vi "_API_BINANCE_DELETE_CanelAllOpenOrderOnASymbol.vi"(0 "BinanceAPI_.lvclass":refnum<class "BinanceAPI_.lvclass">, 5 "CanelAllOpenOrderOnSymbol":T1={"symbol (BTCUSDT)"="CAKEUSDT", "recvWindow"=5000}, 11 "error in (no error)":errorcluster) -> (4 "BinanceAPI_.lvclass 2":refnum<class "BinanceAPI_.lvclass">, 14 "Body":string, 15 "error out":errorcluster)   [LabVIEW 2022 SP3, in "BinanceAPI_.lvclass"]
doc: "Delete all open orders on symbol"
uses:
  BinanceAPI_.lvclass
  BinanceAPI_.lvclass/BinanceAPI_.ctl
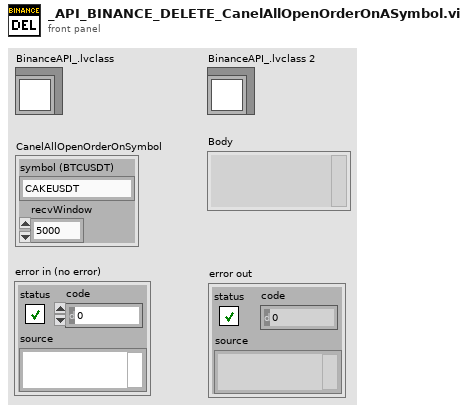
[diagram p1: front panel]
types:
  T1 = cluster{"symbol (BTCUSDT)":string, "recvWindow":i32}
  T2 = enum16{"SPOT", "USDT_FUTURES", "COIN_FUTURES", "VANILLA"}
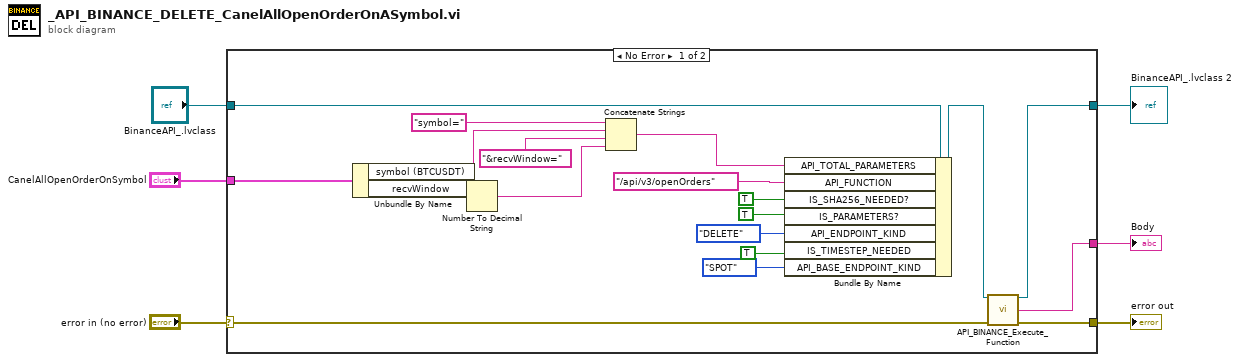
[diagram p0: block diagram]
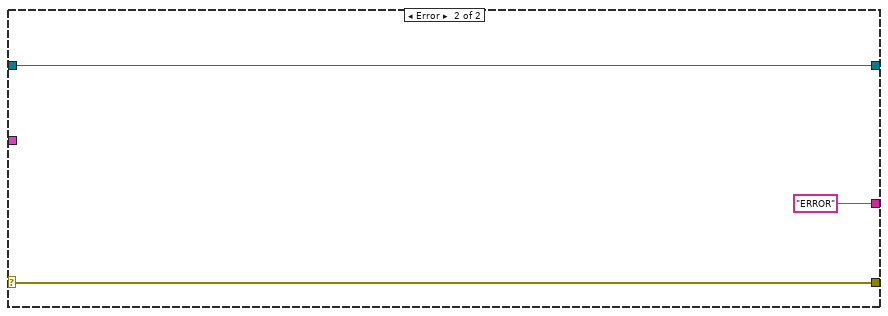
[diagram p2: hidden frame]
diagram:
  n1 = case shown="No Error" "error in (no error)" {
    selector: "error in (no error)" -> [w10 w28]
    tunnel: [w9 w28] -> w5
    tunnel: [w11 w27] -> w1
    tunnel: "BinanceAPI_.lvclass" -> [w19 w27]
    tunnel: "CanelAllOpenOrderOnSymbol" -> [w22 _]
    tunnel: [w8 "ERROR" ("Body")] -> w3
    frame No Error {
      n2 = Unbundle By Name(w22) -> ("symbol (BTCUSDT)"=w15:string, "recvWindow"=w17:i32)
      n3 = Number To Decimal String(number=w17) -> (decimal integer string=w18:string)  [unwired: 1 in]
      n4 = Concatenate Strings("symbol=" ("Symbol"), w15, "&recvWindow=" ("string"), w18) -> (w21:string)
      n5 = Bundle By Name(cluster=w19, "API_TOTAL_PARAMETERS"=w21, "API_FUNCTION"="/api/v3/openOrders", "IS_SHA256_NEEDED?"=TRUE, "IS_PARAMETERS?"=TRUE, "API_ENDPOINT_KIND"=enum16{"POST", "DELETE", "GET", "PUT"}."DELETE", "IS_TIMESTEP_NEEDED"=TRUE, "API_BASE_ENDPOINT_KIND"=T2."SPOT") -> (w12:refnum<class "BinanceAPI_.lvclass">)
      n6 = call "API_BINANCE_Execute_Function.vi"("BinanceAPI in"=w12, "error in (no error)"=w10) -> ("BinanceAPI out"=w11:refnum<class "BinanceAPI_.lvclass">, "Body"=w8:string, "error out"=w9:errorcluster)  [unwired: 9 in, 2 out]
    }
    frame Error {
    }
  }
  "error out" <- w5
  "Body" <- w3
  "BinanceAPI_.lvclass 2" <- w1
